vi "UpdateHistory.vi"(4 "Description":string, 6 "Library":string, 7 "Action":string, 8 "error in (no error)":errorcluster, 9 "ErrorText":string, 10 "ErrorCode":i32, 11 "Connection in":refnum<class "Connection.lvclass">) -> (0 "error out":errorcluster, 3 "Connection out":refnum<class "Connection.lvclass">)   [LabVIEW 2018, in "ErrorDefinitionSQLite.lvclass"]
uses:
  <userlib>/_express/CustomErrorCreator/ErrorDefinitionSQLite/ErrorDefinitionSQLite.lvclass
  <vilib>/drjdpowell/SQLite Library/SQL Connection/Connection.lvclass
  <vilib>/drjdpowell/SQLite Library/SQL Connection/Execute SQL.vi
  <vilib>/drjdpowell/SQLite Library/SQLite.lvlib
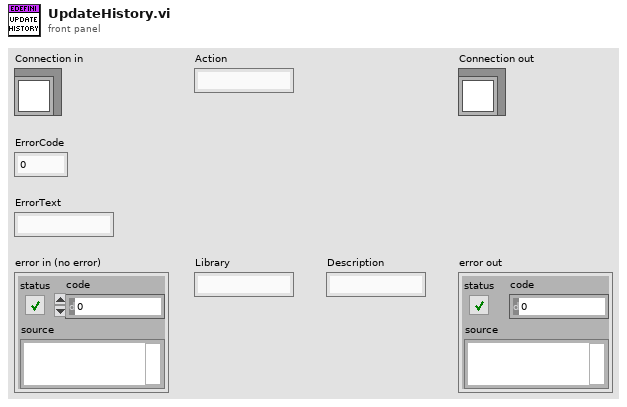
[diagram p1: front panel]
types:
  T1 = cluster{"Action":string, "App.UserName":string, string, "ErrorText":string, "Library":string, "Description":string}
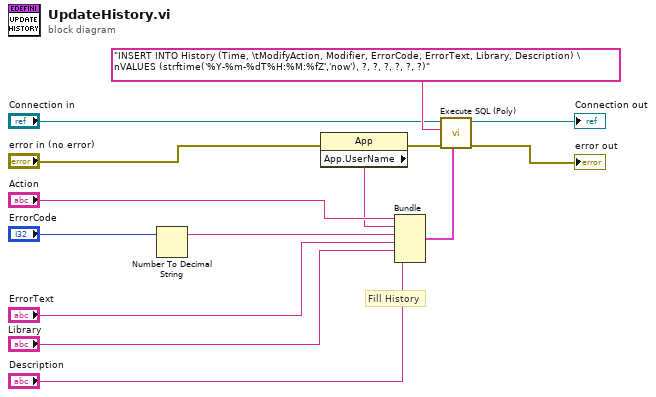
[diagram p0: block diagram]
diagram:
  # "Fill History"
  n1 = Number To Decimal String(number="ErrorCode") -> (decimal integer string=w1:string)  [unwired: 1 in]
  n2 = property class="App"(error in="error in (no error)") -> (error out=w9:errorcluster, "App.UserName"=w6:string)  [unwired: 1 in, 1 out]
  n3 = Bundle("Action"="Action", "App.UserName"=w6, w1, "ErrorText"="ErrorText", "Library"="Library", "Description"="Description") -> (w7:T1)  [unwired: 1 in]
  n4 = call-poly <vilib>:"Execute SQL (Poly).vi"("Parameter(s)"=w7, "error in (no error)"=w9, "SQL"="INSERT INTO History (Time, \tModifyAction, Modifier, ErrorCode, ErrorText, Library, Description) \nVALUES (strftime('%Y-%m-%dT%H:%M:%fZ','now'), ?, ?, ?, ?, ?, ?)", "SQLite Connection in"="Connection in") -> ("error out"=→"error out":errorcluster, "SQLite Connection"=→"Connection out":refnum<class "Connection.lvclass">)  [unwired: 4 in, 2 out]
